vi "Autocycle v0.6.vi"(7 "Message Queue":refnum<queue>, 8 "error in":errorcluster, 10 "All Para":cluster{"Auto Para":T1, "General Para":T2}={"Auto Para"={"Agitator Delays"=[], "TF Delays"=[], "Insertion Delays"=[], "Cutting Delays"=[], "PF Delays"=[], "Measur. Delays"=[], "Reject Delays"=[1000], "BF Delays"=[1000], "P&P Delays"=[1000]}, "General Para"={"Max. Cons."=5.0, "Offset 1"=0.0, "Offset 2"=0.0, "Offset 3"=0.0, "Offset 4"=0.0, "OutputPause"=0.0, "RejectPause"=0.0, "IndexTimeout"=0.0}}, 11 "CleanResume?":bool) -> (0 "error out":errorcluster)   [LabVIEW 2021]
doc: "v0.5:\n- Skip Cutting on frst iteration\n\nv0.3:\n- Added End Cycle & Stop initiated as different stops\n- Make PF & TF not run on the first iteration"
uses:
  support/Message Queue/Message Cluster.ctl
  Controls/Auto Delays.ctl
  support/Controls/General Para.ctl
  Controls/Auto Times.ctl
  Global Variables/RT GV.vi
  Global Variables/FPGA GV.vi
  <vilib>/Utility/error.llb/Error Cluster From Error Code.vi
  <vilib>/rvi/errors/niLvFpgaAdjustHostInterfaceError.vi
  support/Message Queue/Enqueue Message (Single).vi
  <vilib>/rvi/interface/nirviReadWriteControl/nirviReadWriteControl.xnode
  NiFpgaLv.dll
  <vilib>/rvi/interface/Simulation/niFpgaSimulationCallBeginRW.vi
  support/Message Queue/Message Queue.lvlib
panel:
  in  "EnableSOL":bool=TRUE
  out "Iterations to ON":i32
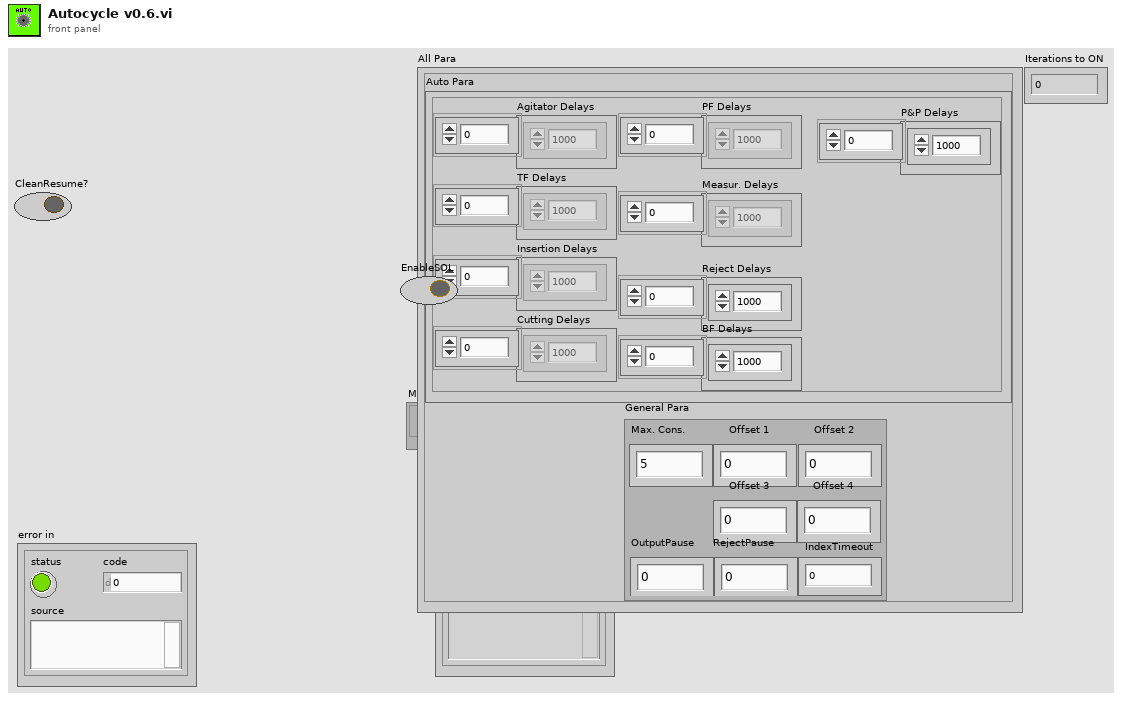
[diagram p1: front panel]
types:
  T1 = typedef "Auto Delays.ctl" = cluster{"Agitator Delays":u32[], "TF Delays":u32[], "Insertion Delays":u32[], "Cutting Delays":u32[], "PF Delays":u32[], "Measur. Delays":dbl[], "Reject Delays":u32[], "BF Delays":u32[], "P&P Delays":u32[]}
  T2 = typedef "General Para.ctl" = cluster{"Max. Cons.":dbl, "Offset 1":dbl, "Offset 2":dbl, "Offset 3":dbl, "Offset 4":dbl, "OutputPause":dbl, "RejectPause":dbl, "IndexTimeout":dbl}
  T3 = cluster{"TL_Red":bool, "TL_Orange":bool, "TL_Green":bool, "TL_Buzzer":bool, "Vaccuum ON":bool, "Vaccuum OFF":bool, "Beckhoff Data":bool, "SOL_Singling":bool, "Bowl Feeder_ ON1":bool, "Buffer 1":bool, "SOL_Pick_Place_Vertical":bool, "SOL_Tube_Feed_Agitatator":bool, "SOL_Tube_Feed_Gating_CYL":bool, "SOL_Insertion _CYL":bool, "SOL_Insertion_Clamp_CYL":bool, "SOL_Cutting_CYL":bool, "SOL_Cutting_Clamp_CYL":bool, "SOL_Insertion_Air_Nozzle":bool, "SOL_Measurement_CYL":bool, "SOL_Pick_Place_Rotary":bool, "SOL_Rejection CYL_1":bool, "SOL_Rejection CYL_2":bool, "SOL_Rejection CYL_3":bool, "SOL_Rejection CYL_4":bool, "Bowl Feeder_ON2":bool, "Linear Feeder 1":bool, "Linear Feeder 2":bool, "Buffer 2":bool, "Buffer 3":bool, "Buffer 4":bool, "Buffer 5":bool, "Buffer 6":bool}
  T4 = typedef "Auto Times.ctl" = cluster{"Index Time":u32, "TF Time":u32, "Insertion Time":u32, "Cutting Time":u32, "PF Time":u32, "Meas. Time":u32, "Reject Time":u32, "P&P Time":u32}
  T5 = cluster{"Reject 1":bool, "Reject 2":bool, "Reject 3":bool, "Reject 4":bool}
  T6 = cluster{"Tube Present":bool[], "Parts Count":u32}
  T7 = cluster{"seconds since 1Jan1904":timestamp, "Auto Times":T4, "Tube Present":bool[], "Reject Pallets":cluster{"Reject 1":bool, "Reject 2":bool, "Reject 3":bool, "Reject 4":bool}, "Measurements":cluster{"1":dbl, "2":dbl, "3":dbl, "4":dbl}}
  T8 = typedef "Auto Stats.ctl" = cluster{"Time-Stamp":timestamp, "Auto Times":T4, "Measurements":cluster{"1":dbl, "2":dbl, "3":dbl, "4":dbl}, "Outputs":cluster{"Good Parts":u32, "Reject Parts":u32}, "Cycle Time":dbl, "Remarks":string}
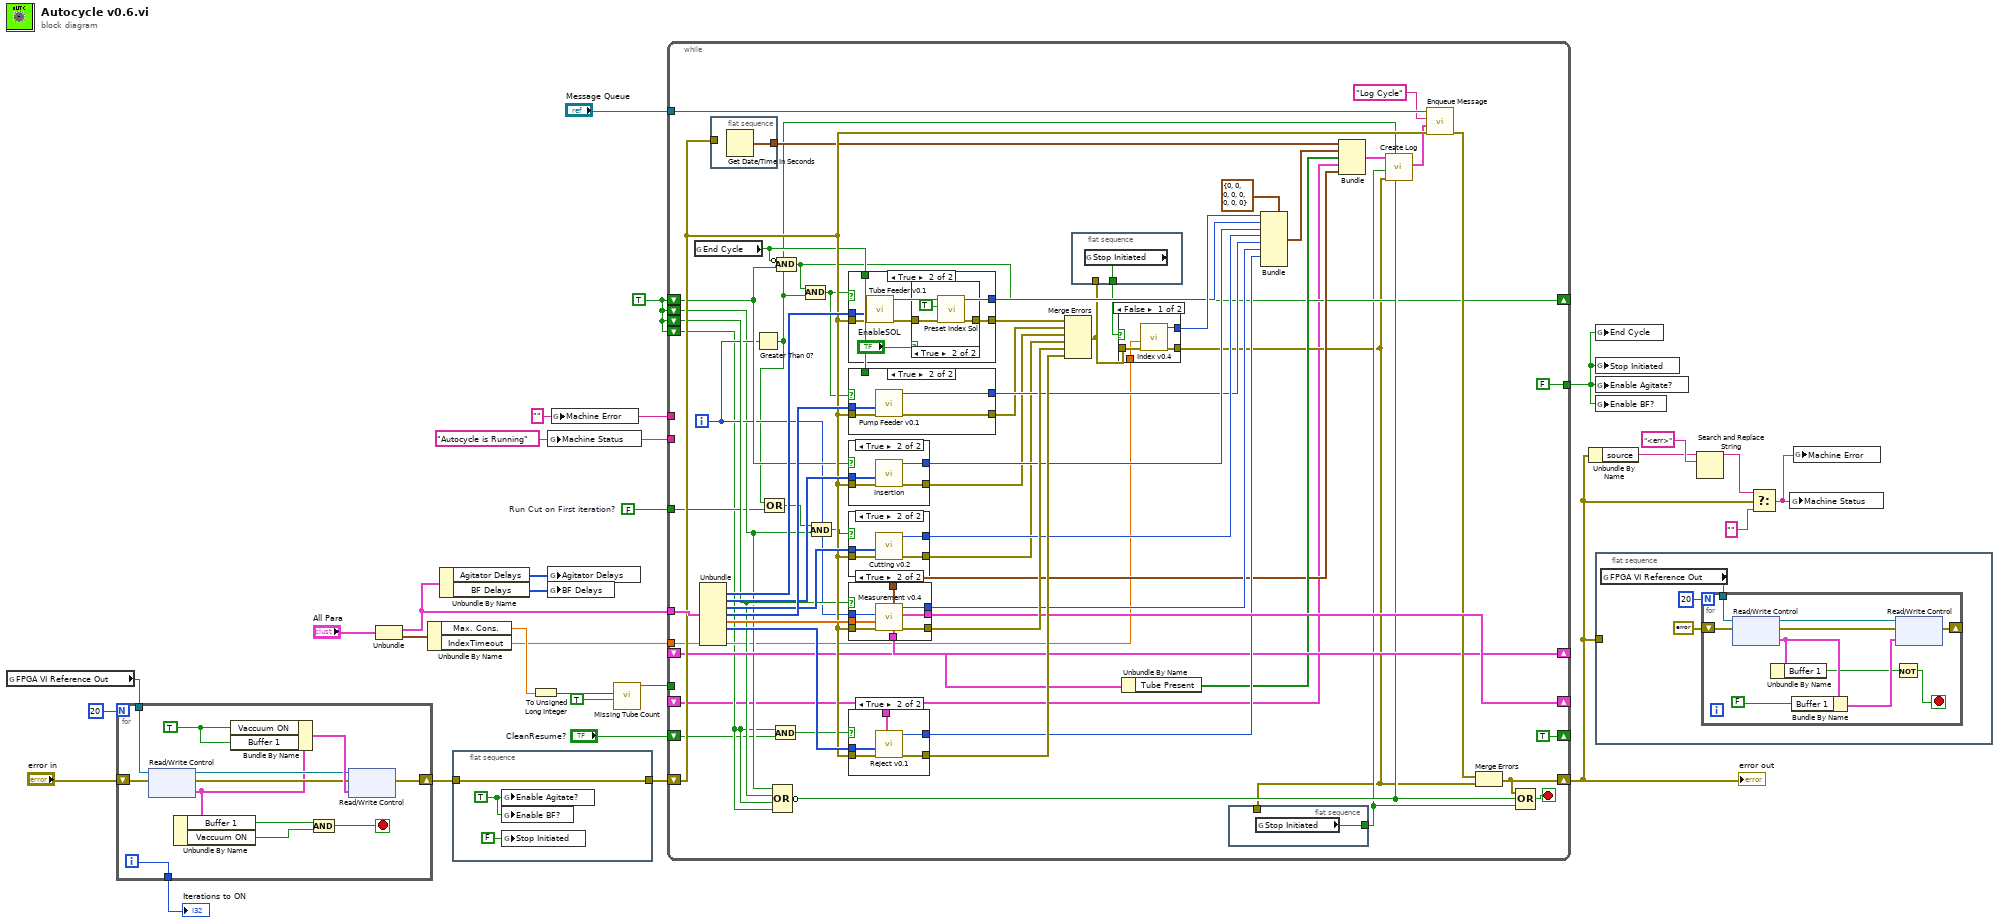
[diagram p0: block diagram]
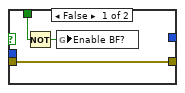
[diagram p3: hidden frame]
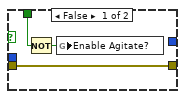
[diagram p6: hidden frame]
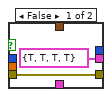
[diagram p9: hidden frame]
diagram:
  w3 = FALSE  # Run Cut on First iteration?
  w17 = "" ("Machine Error")
  w24 = "Autocycle is Running" ("Machine Status")
  w11 = TRUE
  n1 = global read "FPGA GV.vi" "FPGA VI Reference Out"() -> (w27:refnum<k20>)
  n2 = for {
    N: 20 -> [_]
    tunnel: w27 -> [w41]
    shift-right: [w36] -> w14
    shift-left: "error in" -> [w37]
    tunnel: [w30] -> w4
    i -> [w30]
    stop <- w32 stop-if-true
    w33 = TRUE ("Pump_CNVR_Motor _ON")
    n3 = xnode "Read/Write Control"("FPGA VI Reference In"=w41, "error in"=w37) -> ("FPGA VI Reference Out"=w38:refnum<k20>, "error out"=w39:errorcluster, "DO 1"=w35:T3)
    n4 = Unbundle By Name(w35) -> ("Buffer 1"=w34:bool, "Vaccuum ON"=w31:bool)
    n5 = Bundle By Name(cluster=w35, "Vaccuum ON"=w33, "Buffer 1"=w33) -> (w40:T3)
    n6 = Compound Arithmetic op=AND(w34, w31) -> (w32:bool)
    n7 = xnode "Read/Write Control"("FPGA VI Reference In"=w38, "error in"=w39, "DO 1"=w40) -> ("error out"=w36:errorcluster)  [unwired: 1 out]
  }
  "Iterations to ON" <- w4
  n8 = Unbundle("All Para") -> ("Auto Para"=w8:T1, "General Para"=w7:T2)
  n9 = Unbundle By Name(w7) -> ("Max. Cons."=w6:dbl, "IndexTimeout"=w2:dbl)
  n10 = Unbundle By Name(w8) -> ("Agitator Delays"=w29:u32[], "BF Delays"=w28:u32[])
  n11 = flat-sequence {
    tunnel: [w44] -> w13
    tunnel: w14 -> [w44]
    frame #0 {
      w43 = TRUE ("Enable Agitate?")
      n12 = global write "RT GV.vi" "Enable Agitate?"(w43) -> ()
      n13 = global write "RT GV.vi" "Enable BF?"(w43) -> ()
      n14 = global write "RT GV.vi" "Stop Initiated"(FALSE ("Stop Initiated")) -> ()
    }
  }
  n15 = To Unsigned Long Integer(number=w6) -> (unsigned 32bit integer=w5:u32)
  n16 = global write "RT GV.vi" "Machine Status"(w24) -> ()
  n17 = global write "RT GV.vi" "Agitator Delays"(w29) -> ()
  n18 = global write "RT GV.vi" "BF Delays"(w28) -> ()
  n19 = global write "RT GV.vi" "Machine Error"(w17) -> ()
  n20 = call "Missing Tube Count.vi"("ResetMT?"=TRUE, "Max Successive"=w5) -> ("Boolean"=w15:bool)  [unwired: 8 in, 1 out]
  n21 = while {
    tunnel: w8 -> [w99]
    shift-right: [w76] -> w22
    shift-left: w13 -> [w77]
    shift-right: [w93] -> _
    shift-left: _ -> [w45]
    shift-right: [w62] -> _
    shift-left: w11 -> [w63]
    shift-left: w11 -> [w55]
    shift-left: w11 -> [w64]
    shift-left: w11 -> [w49]
    tunnel: "Message Queue" -> [w83]
    tunnel: [FALSE] -> w10
    tunnel: w24 -> [_]
    tunnel: w17 -> [_]
    shift-right: [w71] -> _
    shift-left: _ -> [w70]
    tunnel: w15 -> [_]
    tunnel: w3 -> [w52]
    tunnel: w2 -> [w50]
    shift-right: [TRUE ("ResetMT?")] -> _
    shift-left: "CleanResume?" -> [w47]
    i -> [w59]
    stop <- w92 stop-if-true
    n22 = global read "RT GV.vi" "End Cycle"() -> (w65:bool)
    n23 = Unbundle(w99) -> ("TF Delays"=w102:u32[], "Insertion Delays"=w101:u32[], "Cutting Delays"=w100:u32[], "PF Delays"=w103:u32[], "Measur. Delays"=w97:dbl[], "Reject Delays"=w95:u32[])  [unwired: 3 out]
    n24 = flat-sequence {
      tunnel: w77 -> [_]
      tunnel: [w111] -> w73
      frame #0 {
        n25 = Get Date/Time In Seconds() -> (seconds since 1Jan1904=w111:timestamp)
      }
    }
    n26 = Greater Than 0?(x=w59) -> (x > 0?=w51:bool)
    n27 = Compound Arithmetic op=OR(w51, w52) -> (w53:bool)
    n28 = Compound Arithmetic op=OR(w55, w64, w49, w49) -> (invert w67:bool)
    n29 = Compound Arithmetic op=AND(w49, w47) -> (w48:bool)
    n30 = Compound Arithmetic op=AND(invert w65, w63) -> (w62:bool)
    n31 = Compound Arithmetic op=AND(w62, w51) -> (w61:bool)
    n32 = Compound Arithmetic op=AND(w53, w55) -> (w54:bool)
    n33 = case shown="True" w61 {
      tunnel: w77 -> [w131 w137]
      tunnel: [w131 w133] -> w98
      tunnel: w102 -> [_ w136]
      tunnel: [_ w135] -> w90
      tunnel: w65 -> [w130 _]
      frame False {
        n34 = Not(x=w130) -> (.not. x?=w129:bool)
        n35 = global write "RT GV.vi" "Enable Agitate?"(w129) -> ()
      }
      frame True {
        n36 = call "Tube Feeder v0.1.vi"("error in (no error)"=w137, "TF Para"=w136) -> ("error out"=w134:errorcluster, "TF Time"=w135:u32)  [unwired: 8 in]
        n37 = case shown="True" "EnableSOL" {
          tunnel: w134 -> [w138 w141]
          tunnel: [w138 w140] -> w133
          frame False {
          }
          frame True {
            n38 = call "Preset Index Sol.vi"("error in"=w141, "CCW?"=TRUE) -> ("error out"=w140:errorcluster)  [unwired: 9 in]
          }
        }
      }
    }
    n39 = case shown="True" w61 {
      tunnel: w77 -> [w114 w118]
      tunnel: [w114 w117] -> w79
      tunnel: w103 -> [_ w116]
      tunnel: [_ w115] -> w87
      tunnel: w65 -> [w113 _]
      frame False {
        n40 = Not(x=w113) -> (.not. x?=w112:bool)
        n41 = global write "RT GV.vi" "Enable BF?"(w112) -> ()
      }
      frame True {
        n42 = call "Pump Feeder v0.1.vi"("error in (no error)"=w118, "TF Delays"=w116) -> ("error out"=w117:errorcluster, "PF Time"=w115:u32)  [unwired: 8 in]
      }
    }
    n43 = case shown="True" w63 {
      tunnel: w77 -> [w124 w128]
      tunnel: [w124 w127] -> w80
      tunnel: w101 -> [_ w126]
      tunnel: [_ w125] -> w89
      frame False {
      }
      frame True {
        n44 = call "Insertion.vi"("error in (no error)"=w128, "Insertion Delays"=w126) -> ("error out"=w127:errorcluster, "Insertion Time"=w125:u32)  [unwired: 7 in, 1 out]
      }
    }
    n45 = case shown="True" w54 {
      tunnel: w77 -> [w119 w123]
      tunnel: [w119 w122] -> w81
      tunnel: w100 -> [_ w121]
      tunnel: [_ w120] -> w88
      frame False {
      }
      frame True {
        n46 = call "Cutting v0.2.vi"("error in (no error)"=w123, "Cutting Delays"=w121) -> ("error out"=w122:errorcluster, "Cutting Time"=w120:u32)  [unwired: 8 in]
      }
    }
    n47 = case shown="True" w64 {
      tunnel: w77 -> [w149 w157]
      tunnel: [w149 w156] -> w96
      tunnel: w97 -> [_ w155]
      tunnel: [_ w154] -> w86
      tunnel: [_ w153] -> w68
      tunnel: [T5 {"Reject 1"=TRUE, "Reject 2"=TRUE, "Reject 3"=TRUE, "Reject 4"=TRUE} ("Reject Pallets") w152] -> w93
      tunnel: [_ w151] -> w71
      tunnel: w59 -> [_ w150]
      frame False {
      }
      frame True {
        n48 = call "Measurement v0.4.vi"("error in (no error)"=w157, "TF Delays"=w155, "Loop Count"=w150) -> ("error out"=w156:errorcluster, "Reject Pallets"=w152:T5, "PF Time"=w154:u32, "Part Count"=w151:T6, "Measurements"=w153:cluster{"1":dbl, "2":dbl, "3":dbl, "4":dbl})  [unwired: 4 in]
      }
    }
    n49 = case shown="True" w48 {
      tunnel: w77 -> [w142 w147]
      tunnel: [w142 w146] -> w94
      tunnel: w95 -> [_ w145]
      tunnel: [_ w144] -> w85
      tunnel: w45 -> [_ w143]
      frame False {
      }
      frame True {
        n50 = call "Reject v0.1.vi"("Reject Pallets"=w143, "error in (no error)"=w147, "TF Delays"=w145) -> ("error out"=w146:errorcluster, "PF Time"=w144:u32)  [unwired: 7 in]
      }
    }
    n51 = Merge Errors(w98, w79, w80, w81, w96, w94) -> (w56:errorcluster)
    n52 = flat-sequence {
      tunnel: [w104] -> w57
      tunnel: w56 -> [_]
      frame #0 {
        n53 = global read "RT GV.vi" "Stop Initiated"() -> (w104:bool)
      }
    }
    n54 = case shown="False" w57 {
      tunnel: [w108 _] -> w91
      tunnel: w56 -> [w107 w109]
      tunnel: [w106 w109] -> w58
      tunnel: w50 -> [w105 _]
      frame False {
        n55 = call "Index v0.4.vi"("error in (no error)"=w107, "timeout"=w105) -> ("error out"=w106:errorcluster, "Index Time"=w108:u32)  [unwired: 5 in, 3 out]
      }
      frame True {
      }
    }
    n56 = Unbundle By Name(w70) -> ("Tube Present"=w69:bool[])
    n57 = flat-sequence {
      tunnel: [w110] -> w60
      tunnel: w58 -> [_]
      frame #0 {
        n58 = global read "RT GV.vi" "Stop Initiated"() -> (w110:bool)
      }
    }
    n59 = Bundle(cluster=T4 {"Index Time"=0, "TF Time"=0, "Insertion Time"=0, "Cutting Time"=0, "PF Time"=0, "Meas. Time"=0, "Reject Time"=0, "P&P Time"=0} ("Auto Times"), "Index Time"=w91, "TF Time"=w90, "Insertion Time"=w89, "Cutting Time"=w88, "PF Time"=w87, "Meas. Time"=w86, "Reject Time"=w85) -> (w72:T4)  [unwired: 1 in]
    n60 = Bundle("seconds since 1Jan1904"=w73, "Auto Times"=w72, "Tube Present"=w69, "Reject Pallets"=w45, "Measurements"=w68) -> (w66:T7)  [unwired: 1 in]
    n61 = call "Create Log.vi"("End Cycle?"=w67, "Not First Run?"=w51, "Error in"=w58, "Stop Initiated?"=w60, "Log Input Data"=w66) -> ("Auto Stats"=w74:T8)  [unwired: 6 in]
    n62 = call-poly "Enqueue Message.vi"("error in (no error)"=w77, "Message Data"=w74, "Message"="Log Cycle", "Message Queue"=w83) -> ("error out"=w75:errorcluster)  [unwired: 6 in, 1 out]
    n63 = Merge Errors(w75, w58) -> (w76:errorcluster)
    n64 = Compound Arithmetic op=OR(w76, w67, w60) -> (w92:bool)
  }
  "error out" <- w22
  n65 = Unbundle By Name(w22) -> ("source"=w20:string)
  n66 = global write "RT GV.vi" "End Cycle"(w10) -> ()
  n67 = global write "RT GV.vi" "Stop Initiated"(w10) -> ()
  n68 = global write "RT GV.vi" "Enable Agitate?"(w10) -> ()
  n69 = global write "RT GV.vi" "Enable BF?"(w10) -> ()
  n70 = flat-sequence {
    tunnel: w22 -> [_]
    frame #0 {
      n71 = global read "FPGA GV.vi" "FPGA VI Reference Out"() -> (w159:refnum<k20>)
      n72 = for {
        N: 20 -> [_]
        tunnel: w159 -> [w170]
        shift-right: [w164] -> _
        shift-left: errorcluster {"status"=FALSE, "code"=0, "source"=""} ("error out") -> [w165]
        stop <- w161 stop-if-true
        n73 = xnode "Read/Write Control"("FPGA VI Reference In"=w170, "error in"=w165) -> ("FPGA VI Reference Out"=w166:refnum<k20>, "error out"=w167:errorcluster, "DO 1"=w163:T3)
        n74 = Unbundle By Name(w163) -> ("Buffer 1"=w162:bool)
        n75 = Bundle By Name(cluster=w163, "Buffer 1"=FALSE ("Pump_CNVR_Motor _ON")) -> (w169:T3)
        n76 = Not(x=w162) -> (.not. x?=w161:bool)
        n77 = xnode "Read/Write Control"("FPGA VI Reference In"=w166, "error in"=w167, "DO 1"=w169) -> ("error out"=w164:errorcluster)  [unwired: 1 out]
      }
    }
  }
  n78 = Search and Replace String(input string=w20, search string="<err>") -> (result string=w19:string)  [unwired: 6 in, 3 out]
  n79 = Select(t=w19, s=w22, f="" ("Machine Status")) -> (s? t:f=w18:string)
  n80 = global write "RT GV.vi" "Machine Status"(w18) -> ()
  n81 = global write "RT GV.vi" "Machine Error"(w18) -> ()
